vi "Add SLSC Switch Custom Device.vi"(8 "error in (no error)":errorcluster, 10 "Slot Number":i32, 11 "SLSC Chassis Ref":u64) -> (0 "error out":errorcluster, 2 "SLSC Switch Custom Device Ref":T1 format="%.0x", 3 "SLSC Chassis Ref out":u64)   [LabVIEW 2017, in "SLSC Switch Scripting.lvlib"]
uses:
  SLSC Switch Scripting.lvlib
  <vilib>/NI Veristand/Custom Device API/Custom Device Item Ref.ctl
  NationalInstruments.VeriStand.SystemStorage
  SLSC Scripting Constants.vi
  VeriStand SLSC Scripting/VeriStand SLSC Scripting.lvlib
  <vilib>/NI Veristand/Custom Device API/Custom Device API.lvlib
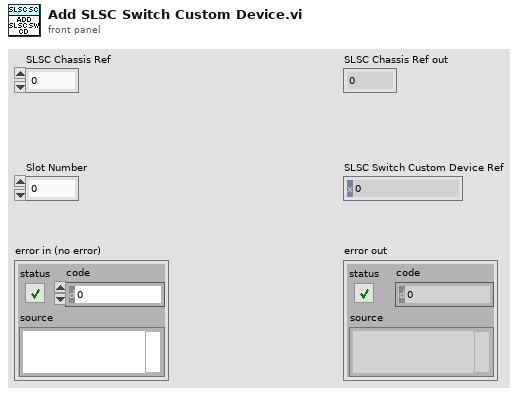
[diagram p1: front panel]
types:
  T1 = typedef "Custom Device API.lvlib/Custom Device Item Ref.ctl" = u64
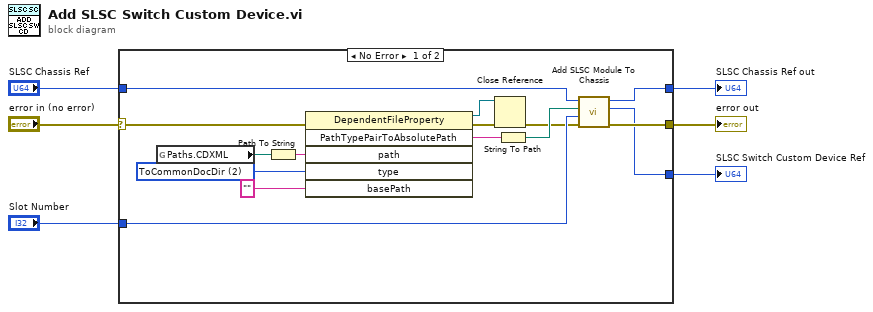
[diagram p0: block diagram]
diagram:
  n1 = case shown="No Error" "error in (no error)" {
    selector: "error in (no error)" -> [w10 w22]
    tunnel: "SLSC Chassis Ref" -> [w15 _]
    tunnel: [w14 _] -> w5
    tunnel: "Slot Number" -> [w13 _]
    tunnel: [w12 w22] -> w3
    tunnel: [w11 _] -> w1
    frame No Error {
      w21 = 2 items=["Absolute", "Relative", "ToCommonDocDir", "ToApplicationDataDir"] ("type")
      n2 = global read "SLSC Scripting Constants.vi" "Paths.CDXML"() -> (w17:path)
      n3 = Path To String(path=w17) -> (string=w19:string)
      n4 = invoke class="DependentFileProperty" method="PathTypePairToAbsolutePath"(error in=w10, "path"=w19, "type"=w21, "basePath"="") -> (reference out=w7:refnum<k24>, error out=w9:errorcluster, "PathTypePairToAbsolutePath"=w18:string)  [unwired: 2 in, 3 out]
      n5 = Close Reference(reference=w7, error in (no error)=w9) -> (error out=w8:errorcluster)
      n6 = String To Path(string=w18) -> (path=w16:path)
      n7 = call "Add SLSC Module To Chassis.vi"("error in (no error)"=w8, "Slot Number"=w13, "SLSC Custom Device XML"=w16, "SLSC Chassis"=w15) -> ("error out"=w12:errorcluster, "SLSC Module"=w11:u64, "SLSC Chassis out"=w14:u64)  [unwired: 5 in]
    }
    frame Error {
    }
  }
  "SLSC Chassis Ref out" <- w5
  "error out" <- w3
  "SLSC Switch Custom Device Ref" <- w1
